vi "cvfilter.vi"() -> ()   [LabVIEW 2020]
uses:
  libs/x86/cvlabview.dll
panel:
  in  "thresh_val":i32
  out "InpImg":T1(plugin-control)
  out "width":dbl
  out "height":dbl
  in  "inpfile":path
  out "OutputIm":T1(plugin-control)
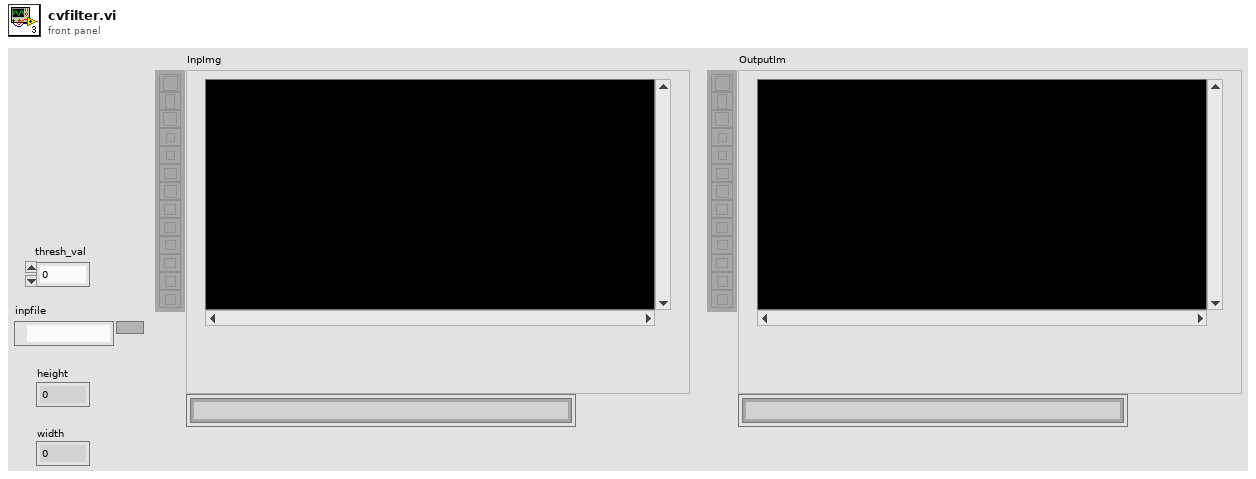
[diagram p1: front panel]
types:
  T1 = typedef "IMAQ Image.ctl" = refnum<image>
  T2 = typedef "Image Type" = u32
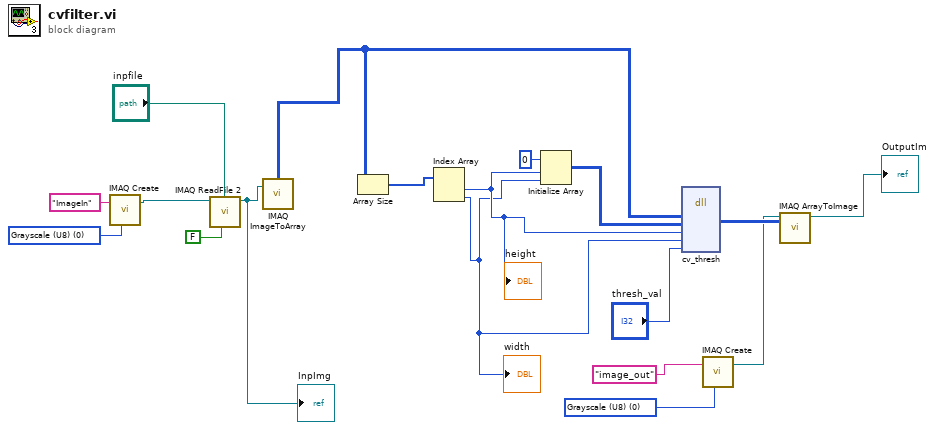
[diagram p0: block diagram]
diagram:
  w7 = T2 0 items=["Grayscale (U8)", "Grayscale (I16)", "Grayscale (SGL)", "Complex (CSG)", "RGB (U32)", "HSL (U32)", "RGB (U64)", "Grayscale (U16)"] ("Image Type")
  w17 = T2 0 items=["Grayscale (U8)", "Grayscale (I16)", "Grayscale (SGL)", "Complex (CSG)", "RGB (U32)", "HSL (U32)", "RGB (U64)", "Grayscale (U16)"] ("Image Type")
  n1 = call "IMAQ Create"("Image Name"="ImageIn", "Image Type"=w17) -> ("New Image"=w16:T1)  [unwired: 3 in, 1 out]
  n2 = call "IMAQ ReadFile 2"("Use File Path Image Type"=FALSE, "File Path"="inpfile", "Image"=w16) -> ("Image Out"=w5:T1)  [unwired: 4 in, 4 out]
  "InpImg" <- w5
  n3 = call "IMAQ ImageToArray"("Image"=w5) -> ("Image Pixels (U8)"=w13:u8[][])  [unwired: 3 in, 4 out]
  n4 = Array Size(array=w13) -> (size(s)=w11:i32[])
  n5 = Index Array(array=w11) -> (element #1=w3:i32, element #2=w2:i32)  [unwired: 2 in]
  "height" <- w3
  "width" <- w2
  n6 = Initialize Array(u8 0 ("element"), w3, w2) -> (w4:u8[][])
  n7 = dll-call lib="C:/Users/shubh/source/repos/cvlabview/vision_filter/libs/x86/cvlabview.dll" fn="cv_thresh"("img_in"=w13, "img_out"=w4, "height"=w3, "width"=w2, "thresh_val"="thresh_val") -> ("img_out"=w14:u8[][])  [unwired: 8 in, 2 out]
  n8 = call "IMAQ Create"("Image Name"="image_out", "Image Type"=w7) -> ("New Image"=w6:T1)  [unwired: 3 in, 1 out]
  n9 = call "IMAQ ArrayToImage"("Image Pixels (U8)"=w14, "Image"=w6) -> ("Image Out"=→"OutputIm":T1)  [unwired: 8 in, 1 out]
